vi "Read Name.vi"(8 "error in (no error)":errorcluster, 11 "Generic Driver in":refnum<class "Generic Driver.lvclass">) -> (0 "error out":errorcluster, 2 "Name":string, 3 "Generic Driver out":refnum<class "Generic Driver.lvclass">)   [LabVIEW 2020, in "OOP.lvlib" / "Generic Driver.lvclass"]
uses:
  Generic Driver.lvclass
  Generic Driver.lvclass/Generic Driver.ctl
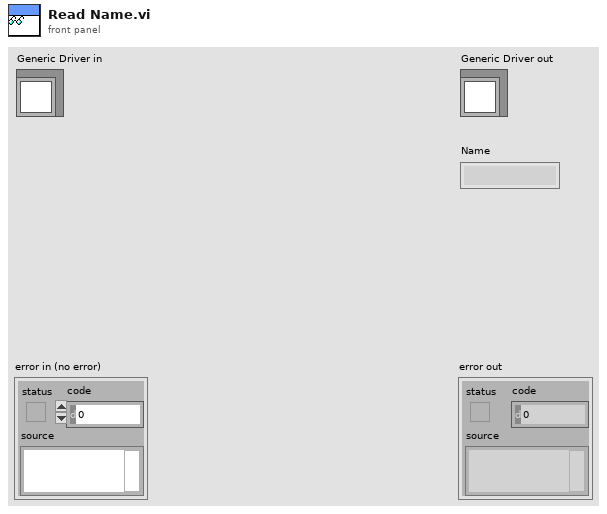
[diagram p1: front panel]
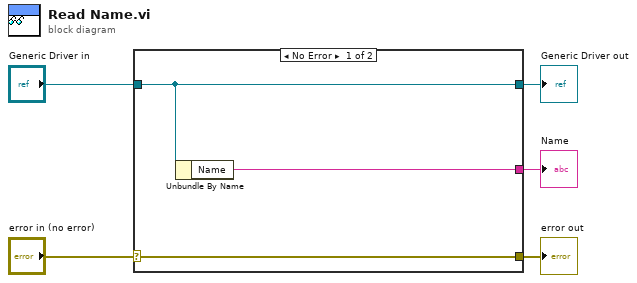
[diagram p0: block diagram]
diagram:
  n1 = case shown="No Error" "error in (no error)" {
    selector: "error in (no error)" -> [w8 w9]
    tunnel: [w8 w9] -> w4
    tunnel: [w7 w10] -> w2
    tunnel: "Generic Driver in" -> [w7 w10]
    tunnel: [w6 _] -> w1
    frame No Error {
      n2 = Unbundle By Name(w7) -> ("Name"=w6:string)
    }
    frame Error {
    }
  }
  "error out" <- w4
  "Generic Driver out" <- w2
  "Name" <- w1
